vi "GEA3 Mix Valve Step Offset Data.vi"(8 "Error In":errorcluster, 11 "MIX VALVE STEP OFFSET (0x400A)":i16) -> (0 "Error Out":errorcluster, 3 "Conv Message Out":string)   [LabVIEW 2019]
uses:
  library/GEA2_Toolkit.lvlib
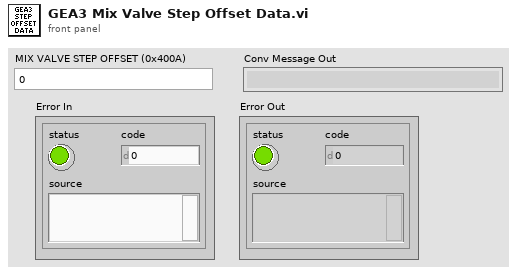
[diagram p1: front panel]
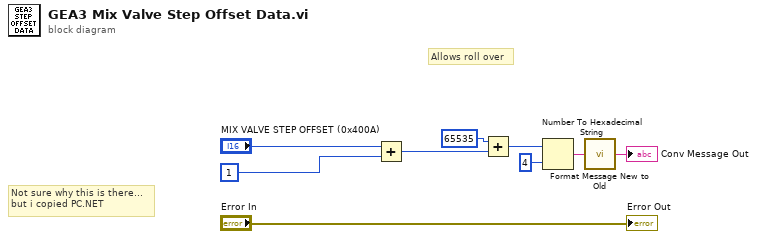
[diagram p0: block diagram]
diagram:
  # "Allows roll over"
  # "Not sure why this is there...\nbut i copied PC.NET"
  n1 = Add(x="MIX VALVE STEP OFFSET (0x400A)", y=u8 1) -> (x+y=w1:i16)
  n2 = Add(x=u16 65535, y=w1) -> (x+y=w9:u16)
  n3 = Number To Hexadecimal String(1:i16 4 ("width (-)"), 2:w9) -> (0:w6:string)
  n4 = call "Format Message New to Old.vi"("Raw Message In"=w6) -> ("Conv Message Out"=→"Conv Message Out":string)  [unwired: 14 in]
  "Error Out" <- "Error In"
